vi "Set_Array of Commands.vi"(8 "error in (no error)":errorcluster, 10 "Array of Commands":T1(array[ring]), 11 "ExampleStateMachine runtime in":refnum<class "ExampleStateMachine runtime.lvclass">) -> (0 "error out":errorcluster, 3 "ExampleStateMachine runtime out":refnum<class "ExampleStateMachine runtime.lvclass">)   [LabVIEW 2017, in "ExampleStateMachine runtime.lvclass"]
uses:
  ExampleStateMachine runtime.lvclass
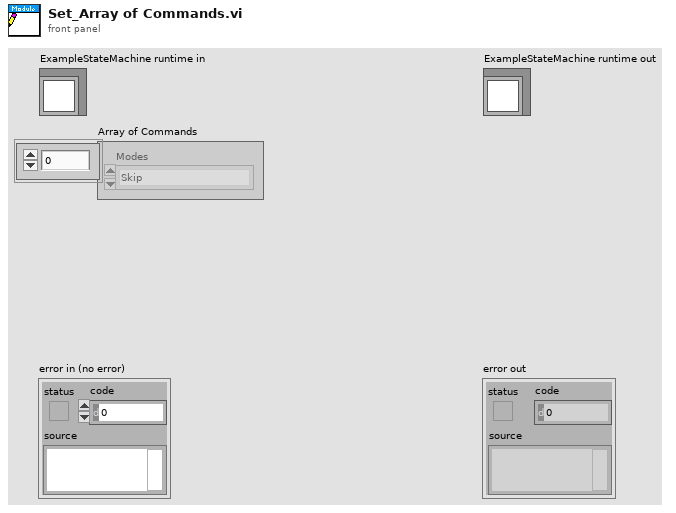
[diagram p1: front panel]
types:
  T1 = enum16{"Reserved", "Profile Position Mode", "Velocity Mode", "Profile Velocity Mode", "Profile Torque Mode", "Reserved 2", "Reference Mode", "Interpolated Position Mode", "Skip"}[]
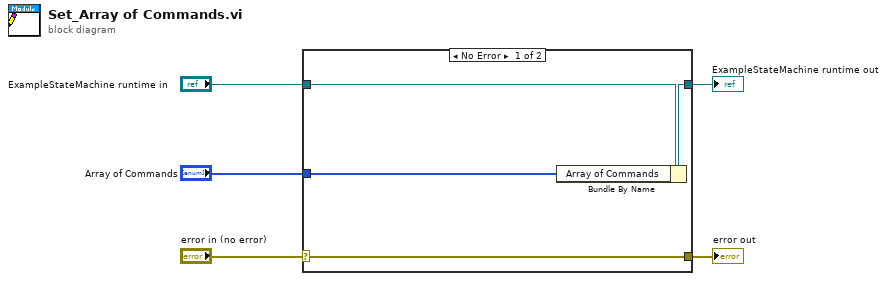
[diagram p0: block diagram]
diagram:
  n1 = case shown="No Error" "error in (no error)" {
    selector: "error in (no error)" -> [w9 w10]
    tunnel: [w9 w10] -> w4
    tunnel: [w7 w11] -> w2
    tunnel: "ExampleStateMachine runtime in" -> [w8 w11]
    tunnel: "Array of Commands" -> [w6 _]
    frame No Error {
      n2 = Bundle By Name(cluster=w8, "Array of Commands"=w6) -> (w7:refnum<class "ExampleStateMachine runtime.lvclass">)
    }
    frame Error {
    }
  }
  "error out" <- w4
  "ExampleStateMachine runtime out" <- w2
